vi "Configure Marker Search.vi"(7 "Marker Search":T1(ring), 8 "error in (no error)":errorcluster, 9 "Target Value":dbl, 10 "Marker Number":u8=1, 11 "VNA-CMT S2 S4 in":refnum<class "VNA-CMT S2 S4.lvclass">) -> (0 "error out":errorcluster, 3 "VNA-CMT S2 S4 out":refnum<class "VNA-CMT S2 S4.lvclass">)   [LabVIEW 2020, in "VNA-CMT S2 S4.lvclass"]
doc: "Configures and excecutes a marker search.\nThe marker is on the active trace."
uses:
  VNA-CMT S2 S4.lvclass
  C:/Sandbox/Git_Sandbox/WiSpry Test Framework source code (LV20)/WiSpry Test Framework/Instruments/Instrument.lvclass
  Instrument.lvclass/Instrument.ctl
  Instrument.lvclass
  <instrlib>/CMT S2 and S4 VNA/CMT S2 and S4 VNA.lvlib
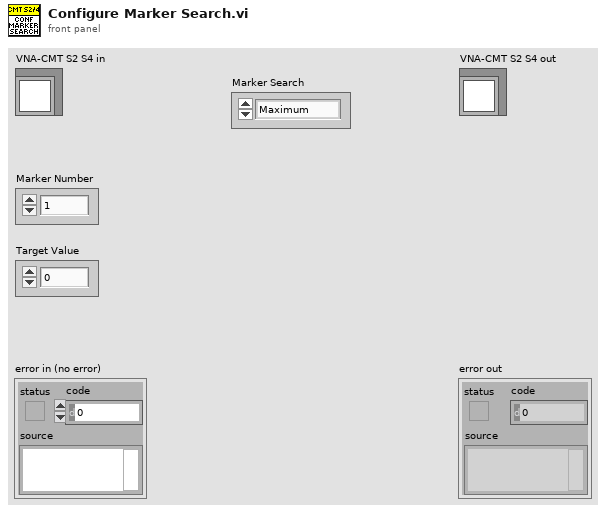
[diagram p1: front panel]
types:
  T1 = enum16{"Maximum", "Minimum", "Right Peak", "Left Peak", "Negative Peak", "Taget Value", "Left Taget Value", "Rigth Target Value"}
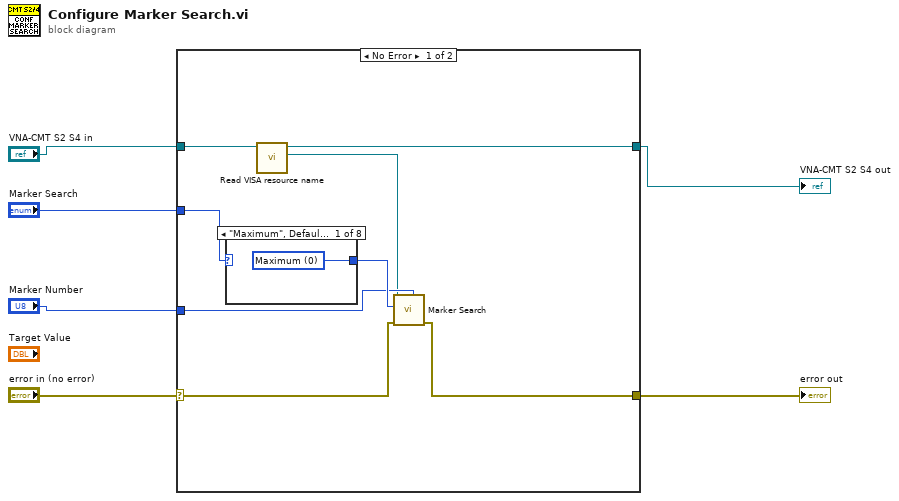
[diagram p0: block diagram]
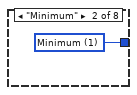
[diagram p2: hidden frame]
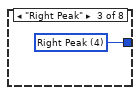
[diagram p3: hidden frame]
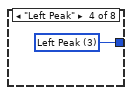
[diagram p4: hidden frame]
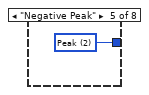
[diagram p5: hidden frame]
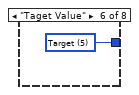
[diagram p6: hidden frame]
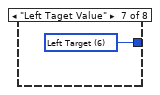
[diagram p7: hidden frame]
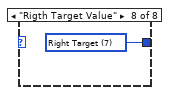
[diagram p8: hidden frame]
diagram:
  n1 = case shown="No Error" "error in (no error)" {
    selector: "error in (no error)" -> [w10 w23]
    tunnel: "VNA-CMT S2 S4 in" -> [w14 w24]
    tunnel: [w13 w24] -> w3
    tunnel: [w8 w23] -> w5
    tunnel: "Marker Search" -> [w12 _]
    tunnel: "Marker Number" -> [w9 _]
    frame No Error {
      n2 = case shown="\"Maximum\", Default" w12 {
        tunnel: [w15 w16 w17 w18 w19 w20 w21 w22] -> w11
        frame "Maximum", Default {
          w15 = u16 0 items=["Maximum", "Minimum", "Peak", "Left Peak", "Right Peak", "Target", "Left Target", "Right Target"] ("Function (0: Maximum)")
        }
        frame "Minimum" {
          w16 = u16 1 items=["Maximum", "Minimum", "Peak", "Left Peak", "Right Peak", "Target", "Left Target", "Right Target"] ("Function (0: Maximum)")
        }
        frame "Right Peak" {
          w17 = u16 4 items=["Maximum", "Minimum", "Peak", "Left Peak", "Right Peak", "Target", "Left Target", "Right Target"] ("Function (0: Maximum)")
        }
        frame "Left Peak" {
          w18 = u16 3 items=["Maximum", "Minimum", "Peak", "Left Peak", "Right Peak", "Target", "Left Target", "Right Target"] ("Function (0: Maximum)")
        }
        frame "Negative Peak" {
          w19 = u16 2 items=["Maximum", "Minimum", "Peak", "Left Peak", "Right Peak", "Target", "Left Target", "Right Target"] ("Function (0: Maximum)")
        }
        frame "Taget Value" {
          w20 = u16 5 items=["Maximum", "Minimum", "Peak", "Left Peak", "Right Peak", "Target", "Left Target", "Right Target"] ("Function (0: Maximum)")
        }
        frame "Left Taget Value" {
          w21 = u16 6 items=["Maximum", "Minimum", "Peak", "Left Peak", "Right Peak", "Target", "Left Target", "Right Target"] ("Function (0: Maximum)")
        }
        frame "Rigth Target Value" {
          w22 = u16 7 items=["Maximum", "Minimum", "Peak", "Left Peak", "Right Peak", "Target", "Left Target", "Right Target"] ("Function (0: Maximum)")
        }
      }
      n3 = call "Read VISA resource name.vi"("Instrument in"=w14) -> ("VISA resource name"=w7:refnum<visa-resource-name>, "Instrument out"=w13:refnum<class "VNA-CMT S2 S4.lvclass">)  [unwired: 9 in]
      n4 = call <instrlib>:"Marker Search.vi"("Marker (1)"=w9, "error in (no error)"=w10, "Function (0: Maximum)"=w11, "VISA resource name"=w7) -> ("error out"=w8:errorcluster)  [unwired: 3 in, 4 out]
    }
    frame Error {
    }
  }
  "error out" <- w5
  "VNA-CMT S2 S4 out" <- w3
